vi "Error Processor.vi"(8 "error in (no error)":errorcluster, 11 "arsnars in":refnum<class "test_us.lvclass">) -> (0 "error out":errorcluster, 3 "arsnars out":refnum<class "test_us.lvclass">)   [LabVIEW 2026, in "test_us.lvlib" / "test_us.lvclass"]
doc: "Use this VI to process all the error that are solvable inside this specific uService. Whatever is not possible to process, let it leave this VI and it will be processed by the Error Manager of the Distributed System."
uses:
  test_us.lvclass
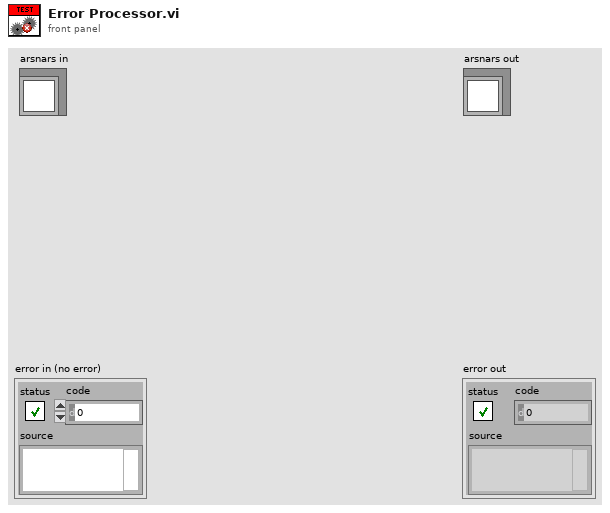
[diagram p1: front panel]
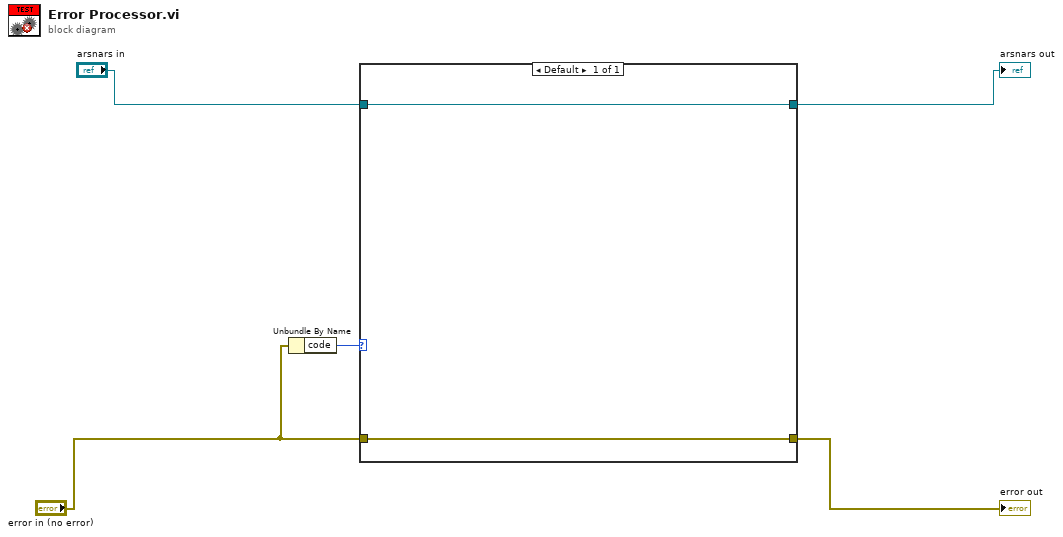
[diagram p0: block diagram]
diagram:
  n1 = Unbundle By Name("error in (no error)") -> ("code"=w1:i32)
  n2 = case shown="Default" w1 {
    tunnel: "error in (no error)" -> [w7]
    tunnel: [w7] -> w5
    tunnel: "arsnars in" -> [w6]
    tunnel: [w6] -> w4
    frame Default {
    }
  }
  "error out" <- w5
  "arsnars out" <- w4
